vi "Start User Interface for Application.vi"(4 "Status References":refnum<vi>[](array[refnum]), 6 "Serial References":refnum<vi>[](array[refnum]), 9 "Test Information":refnum<vi>, 10 "Name":string, 11 "Application in":refnum<class "Application.lvclass">) -> (0 "error out":errorcluster, 3 "Application out":refnum<class "Application.lvclass">)   [LabVIEW 2017, in "Application.lvlib" / "Application.lvclass"]
doc: "Creates the application class, bundles the front panel references into it, and starts all the appropriate processes and classes."
uses:
  Application.lvclass
  C:/Program Files (x86)/National Instruments/LabVIEW 2017/vi.lib/TSS/ACRObat Test Framework/Classes/Base Objects/Base Class/Base Class/Base Class.lvclass
  <vilib>/TSS/ACRObat Test Framework/Classes/Base Objects/Base Class/Base Class/Base Class.lvclass
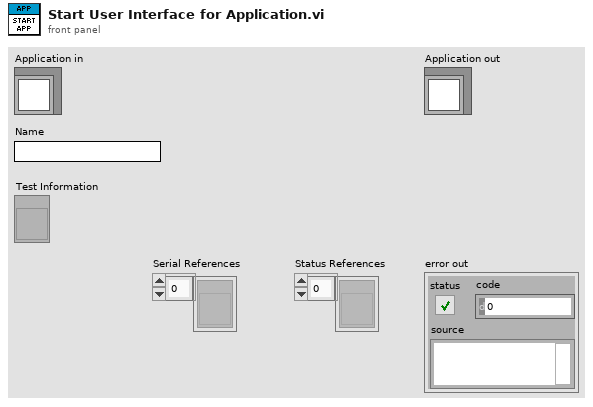
[diagram p1: front panel]
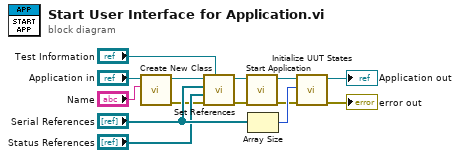
[diagram p0: block diagram]
diagram:
  n1 = call <vilib>:"Create New Class.vi"("Name"="Name", "Base Class in"="Application in") -> ("error out"=w5:errorcluster, "Base Class out"=w7:refnum<class "Application.lvclass">)  [unwired: 8 in]
  n2 = call "Set References.vi"("Test Information"="Test Information", "error in (no error)"=w5, "Status References"="Status References", "Serial References"="Serial References", "Acrobat Template in"=w7) -> ("error out"=w3:errorcluster, "Acrobat Template out"=w4:refnum<class "Application.lvclass">)  [unwired: 5 in]
  n3 = call "Start Application.vi"("error in (no error)"=w3, "Application in"=w4) -> ("error out"=w12:errorcluster, "Application out"=w13:refnum<class "Application.lvclass">)  [unwired: 8 in]
  n4 = Array Size(array="Serial References") -> (size(s)=w14:i32)
  n5 = call-dynamic "Initialize UUT States.vi"("error in (no error)"=w12, "Number of UUTs"=w14, "Application in"=w13) -> ("error out"=→"error out":errorcluster, "Application out"=→"Application out":refnum<class "Application.lvclass">)  [unwired: 7 in]
